vi "Hack Map into JSON.vi"(5 "Value":variant, 7 "Name":string, 11 "JSON in":string) -> (3 "JSON out":string)   [LabVIEW 2023]
uses:
  <vilib>/regexp/Match Regular Expression.xnode
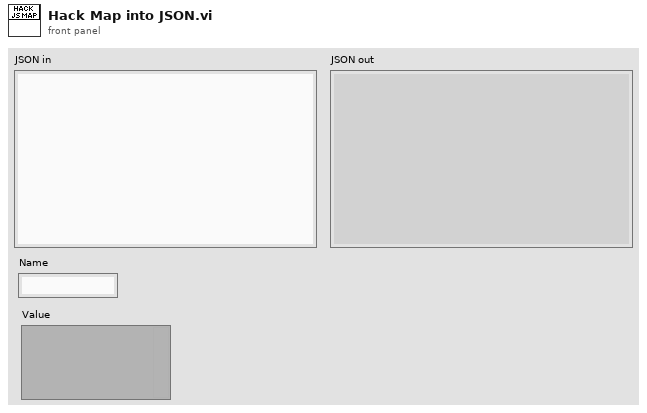
[diagram p1: front panel]
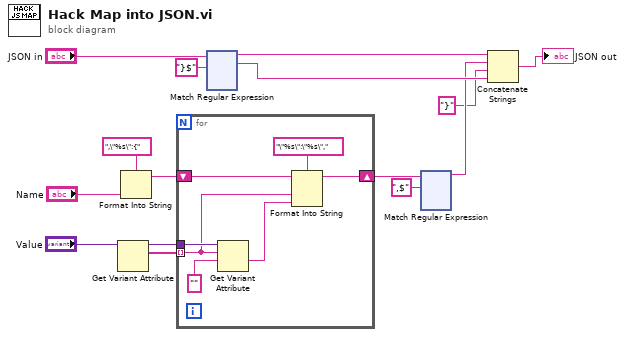
[diagram p0: block diagram]
diagram:
  n1 = Get Variant Attribute(Variant="Value") -> (duplicate Variant=w9:variant, names=w8:string[])  [unwired: 3 in, 2 out]
  n2 = Format Into String(format string=",\"%s\":{" ("regular expression"), "Name") -> (resulting string=w10:string)  [unwired: 2 in, 1 out]
  n3 = for {
    shift-right: [w18] -> w6
    shift-left: w10 -> [w20]
    tunnel: w9 -> [w22]
    tunnel: w8 -> [w17] mode=indexing
    n4 = Get Variant Attribute(Variant=w22, name=w17, default value (empty Variant)="" ("regular expression")) -> (value=w16:string)  [unwired: 1 in, 3 out]
    n5 = Format Into String(format string="\"%s\":\"%s\"," ("regular expression"), initial string=w20, w17, w16) -> (resulting string=w18:string)  [unwired: 1 in, 1 out]
  }
  n6 = xnode "Match Regular Expression"("input string"="JSON in", "regular expression"="}$") -> ("before match"=w5:string, "whole match"=w4:string)  [unwired: 4 in, 3 out]
  n7 = xnode "Match Regular Expression"("input string"=w6, "regular expression"=",$") -> ("before match"=w3:string)  [unwired: 4 in, 4 out]
  n8 = Concatenate Strings(w5, w3, "}" ("regular expression"), w4) -> (→"JSON out":string)
